vi "Init CH Names.vi"(8 "error in (no error)":errorcluster, 11 "Analog-Output in":refnum<class "Analog-Output.lvclass">) -> (0 "error out":errorcluster, 3 "Analog-Output out":refnum<class "Analog-Output.lvclass">)   [LabVIEW 2019, in "Analog-Output.lvlib" / "Analog-Output.lvclass"]
uses:
  Library/Analog-Output.lvclass
  C:/Users/Public/Documents/Development/builds/Tools/Config.lvlibp/Config.lvclass
  Library/Analog-Output.lvclass/Analog-Output.ctl
  Accessors/Write Channel Names.vi
  builds/Tools/Config.lvlibp/Accessors/Read Device Signals.vi
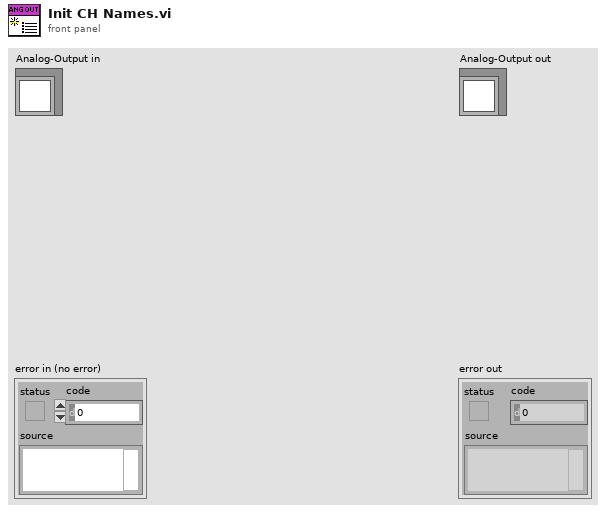
[diagram p1: front panel]
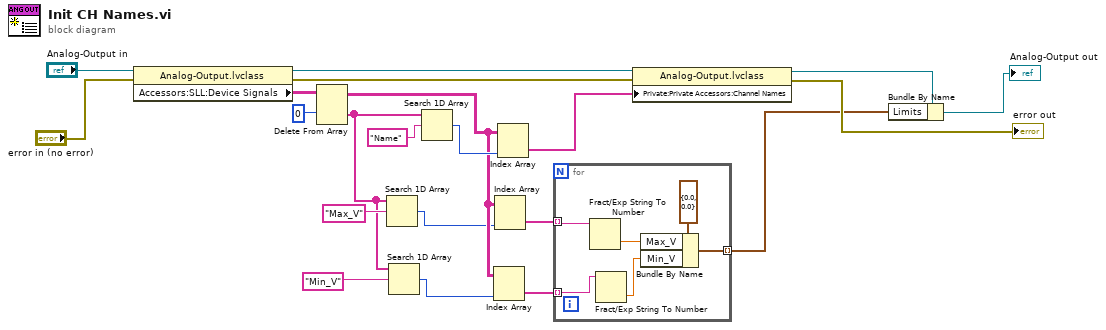
[diagram p0: block diagram]
diagram:
  n1 = property class="Analog-Output.lvclass"(reference="Analog-Output in", error in="error in (no error)") -> (reference out=w15:refnum<class "Analog-Output.lvclass">, error out=w14:errorcluster, "Accessors:SLL:Device Signals"=w18:string[][])
  n2 = Delete From Array(array=w18, index (row)=0 ("disabled index (col)")) -> (deleted portion=w9:string[], array with subset deleted=w8:string[][])  [unwired: 2 in]
  n3 = Search 1D Array(1D array=w9, element="Max_V") -> (index of element=w7:i32)  [unwired: 1 in]
  n4 = Search 1D Array(1D array=w9, element="Min_V") -> (index of element=w6:i32)  [unwired: 1 in]
  n5 = Search 1D Array(1D array=w9, element="Name") -> (index of element=w17:i32)  [unwired: 1 in]
  n6 = Index Array(array=w8, index (col)=w6) -> (element=w2:string[])  [unwired: 1 in]
  n7 = Index Array(array=w8, index (col)=w7) -> (element=w3:string[])  [unwired: 1 in]
  n8 = Index Array(array=w8, index (col)=w17) -> (element=w13:string[])  [unwired: 1 in]
  n9 = for {
    tunnel: w3 -> [w26] mode=indexing
    tunnel: w2 -> [w25] mode=indexing
    tunnel: [w22] -> w1 mode=indexing
    n10 = Fract/Exp String To Number(string=w26) -> (number=w23:dbl)  [unwired: 3 in, 1 out]
    n11 = Fract/Exp String To Number(string=w25) -> (number=w24:dbl)  [unwired: 3 in, 1 out]
    n12 = Bundle By Name(cluster=cluster{"Max_V":dbl, "Min_V":dbl} {"Max_V"=0.0, "Min_V"=0.0} ("Limits"), "Max_V"=w23, "Min_V"=w24) -> (w22:cluster{"Max_V":dbl, "Min_V":dbl})
  }
  n13 = property class="Analog-Output.lvclass"(reference=w15, error in=w14, "Private:Private Accessors:Channel Names"=w13) -> (reference out=w5:refnum<class "Analog-Output.lvclass">, error out=→"error out":errorcluster)
  n14 = Bundle By Name(cluster=w5, "Limits"=w1) -> (→"Analog-Output out":refnum<class "Analog-Output.lvclass">)
